vi "SysDef.UpdateCDVersionFromXML.vi"(8 "error in (no error)":errorcluster, 11 "Device Ref in":T1 format="%.0x") -> (0 "error out":errorcluster, 1 "old version":string, 2 "new version":string, 3 "Device Ref out":T1=18446744073709551615 format="%.0x", 4 "version change?":bool)   [LabVIEW 2024, in "Advanced System Definition.lvlib"]
doc: "This VI checks the version of the Custom Device in the XML, compares it to the version in memory, and updates the version number if they don't match. This VI can be used within a ActionVIOnLoad VI as part of a Custom Device's version migration code."
uses:
  Advanced System Definition.lvlib
  <vilib>/xml/NI_XML.lvlib
  <vilib>/xml/Close Reference(Node).vi
  <vilib>/xml/Load XML File.vi
  <vilib>/xml/XPath/Get First Matched Node (String).vi
  <vilib>/xml/Get Node Text Content (String).vi
  <vilib>/NI VeriStand/Custom Device API/Custom Device Item Ref.ctl
  <vilib>/NI VeriStand/Custom Device API/Custom Device API.lvlib
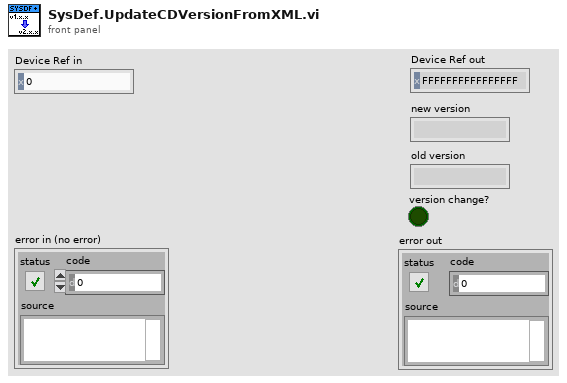
[diagram p1: front panel]
types:
  T1 = typedef "Custom Device API.lvlib/Custom Device Item Ref.ctl" = u64
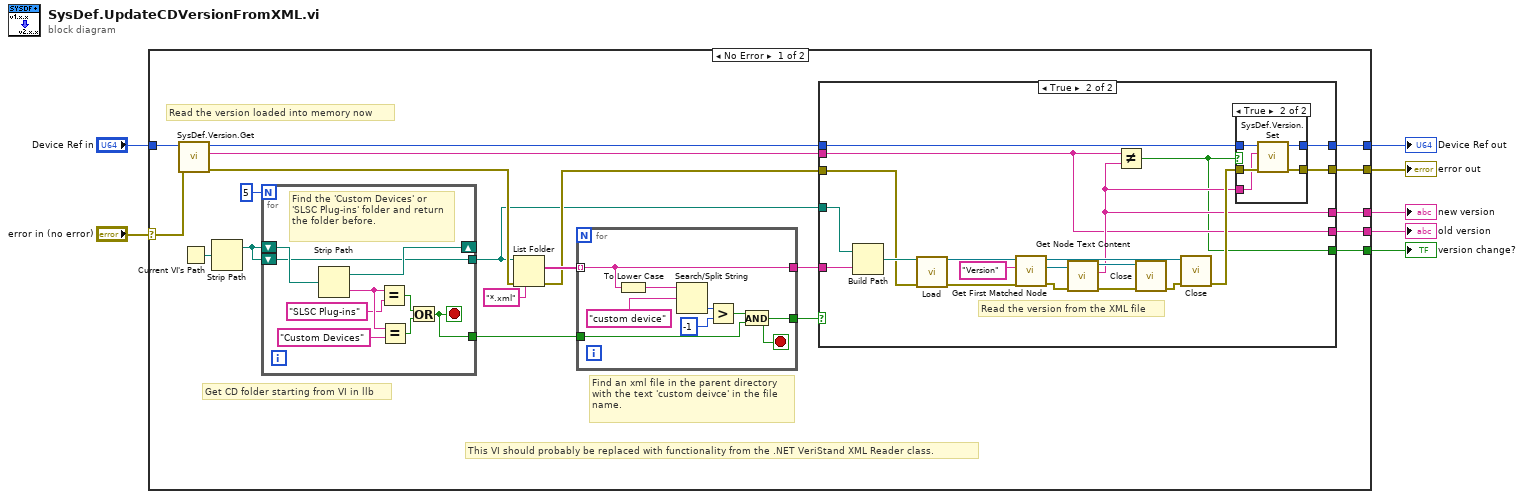
[diagram p0: block diagram]
diagram:
  n1 = case shown="No Error" "error in (no error)" {
    selector: "error in (no error)" -> [w24 w75]
    tunnel: "Device Ref in" -> [w25 w76]
    tunnel: [w17 w76] -> w5
    tunnel: [w16 w75] -> w4
    tunnel: [w15 _] -> w3
    tunnel: [w14 _] -> w2
    tunnel: [w13 _] -> w1
    frame No Error {
      # "This VI should probably be replaced with functionality from the .NET VeriStand XML Reader class."
      # "Read the version loaded into memory now"
      # "Find an xml file in the parent directory with the text 'custom deivce' in the file name."
      # "Get CD folder starting from VI in llb"
      n2 = call "SysDef.Version.Get.vi"("error in (no error)"=w24, "nodeID"=w25) -> ("error out"=w20:errorcluster, "Version"=w8:string, "nodeID out"=w18:u64)  [unwired: 7 in]
      n3 = Current VI's Path() -> (path=w26:path)
      n4 = Strip Path(path=w26) -> (stripped path=w12:path)  [unwired: 1 out]
      n5 = for {
        N: 5 -> [_]
        shift-right: [w35] -> _
        shift-left: w12 -> [w36]
        shift-left: w12 -> [w29]
        tunnel: [w29] -> w10
        tunnel: [w28] -> w9
        stop <- w28 stop-if-true
        # "Find the 'Custom Devices' or 'SLSC Plug-ins' folder and return the folder before."
        n6 = Strip Path(path=w36) -> (stripped path=w35:path, name=w34:string)
        n7 = Equal?(x=w34, y="SLSC Plug-ins") -> (x = y?=w31:bool)
        n8 = Equal?(x=w34, y="Custom Devices") -> (x = y?=w30:bool)
        n9 = Or(x=w31, y=w30) -> (x .or. y?=w28:bool)
      }
      n10 = List Folder(path=w10, pattern="*.xml", error in=w20) -> (filenames=w23:string[], error out=w19:errorcluster)  [unwired: 1 in, 2 out]
      n11 = for {
        tunnel: w23 -> [w74] mode=indexing
        tunnel: [w74] -> w22
        tunnel: [w67] -> w21
        tunnel: w9 -> [w68]
        stop <- w67 stop-if-true
        n12 = To Lower Case(string=w74) -> (all lower case string=w73:string)
        n13 = Search/Split String(string=w73, search string/char (-)="custom device") -> (offset of match=w71:i32)  [unwired: 1 in, 2 out]
        n14 = Greater?(x=w71, y=-1) -> (0:w69:bool)
        n15 = And(x=w69, y=w68) -> (x .and. y?=w67:bool)
      }
      n16 = case shown="True" w21 {
        tunnel: w10 -> [_ w59]
        tunnel: w22 -> [_ w58]
        tunnel: w19 -> [w38 w51]
        tunnel: w18 -> [w39 w46]
        tunnel: w8 -> [w37 w41]
        tunnel: [w39 w44] -> w17
        tunnel: [w38 w43] -> w16
        tunnel: [w37 w42] -> w15
        tunnel: [w37 w41] -> w14
        tunnel: [_ w40] -> w13
        frame False {
        }
        frame True {
          # "Read the version from the XML file"
          n17 = Build Path(base path=w59, name or relative path=w58) -> (appended path=w55:path)
          n18 = call-poly <vilib>:"Load.vi"("path to XML document"=w55, "error in (no error)"=w51) -> ("DOM document out"=w53:refnum<k20>, "error out"=w52:errorcluster)  [unwired: 11 in, 1 out]
          n19 = call-poly <vilib>:"Get First Matched Node.vi"("error in (no error)"=w52, "XPath expression"="Version", "node in"=w53) -> ("error out"=w57:errorcluster, "node result"=w56:refnum<k20>, "node out"=w48:refnum<k20>)  [unwired: 6 in]
          n20 = call-poly <vilib>:"Get Node Text Content.vi"("error in (no error)"=w57, "node in"=w56) -> ("error out"=w49:errorcluster, "node text"=w42:string, "node out"=w50:refnum<k20>)  [unwired: 7 in]
          n21 = Not Equal?(x=w41, y=w42) -> (x != y?=w40:bool)
          n22 = call-poly <vilib>:"Close.vi"("error in (no error)"=w49, "node"=w50) -> ("error out"=w47:errorcluster)  [unwired: 7 in]
          n23 = call-poly <vilib>:"Close.vi"("error in (no error)"=w47, "node"=w48) -> ("error out"=w45:errorcluster)  [unwired: 7 in]
          n24 = case shown="True" w40 {
            tunnel: w46 -> [w61 w66]
            tunnel: w45 -> [w60 w65]
            tunnel: [w60 w64] -> w43
            tunnel: w42 -> [_ w62]
            tunnel: [w61 w63] -> w44
            frame False {
            }
            frame True {
              n25 = call "SysDef.Version.Set.vi"("error in (no error)"=w65, "Version"=w62, "nodeID"=w66) -> ("error out"=w64:errorcluster, "nodeID out"=w63:u64)  [unwired: 7 in]
            }
          }
        }
      }
    }
    frame Error {
    }
  }
  "Device Ref out" <- w5
  "error out" <- w4
  "new version" <- w3
  "old version" <- w2
  "version change?" <- w1
